vi "3Mult.vi"(2 "x3":dbl, 3 "x6":dbl, 4 "x5":dbl, 5 "x4":dbl, 6 "x2":dbl, 7 "x1":dbl) -> (0 "Result":dbl, 1 "Result2":dbl)   [LabVIEW 2025]
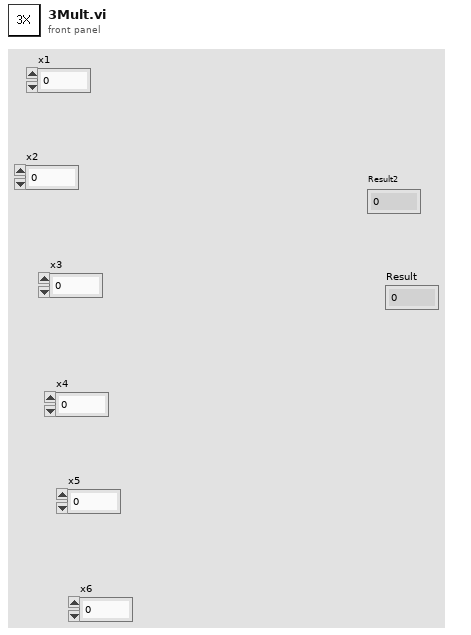
[diagram p1: front panel]
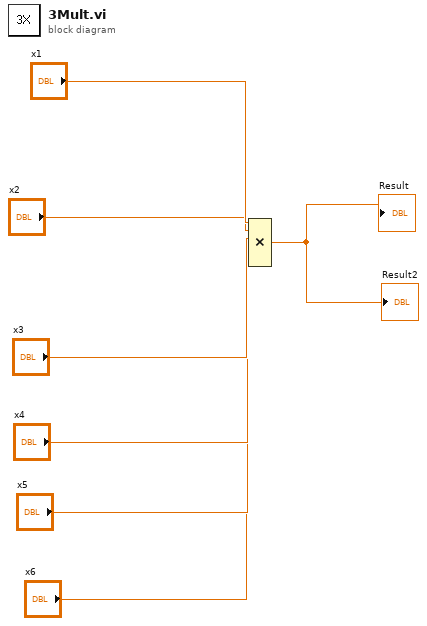
[diagram p0: block diagram]
diagram:
  n1 = Compound Arithmetic op=MULTIPLY("x1", "x2", "x3", "x4", "x5", "x6") -> (→"Result" →"Result2":dbl)
